vi "MRay Auton.vi"(0 "Auton Array":dbl[][](array[numeric])) -> (13 "Shooter":dbl, 14 "Left Drive":dbl, 15 "Right Drive":dbl, 16 "Ramp ACT motor":dbl, 17 "Conveyor":dbl, 18 "Harvester":dbl, 19 "Turret Rotation":dbl)   [LabVIEW 2011]
uses:
  Robot Global Data.vi
panel:
  out "Tzero":i64
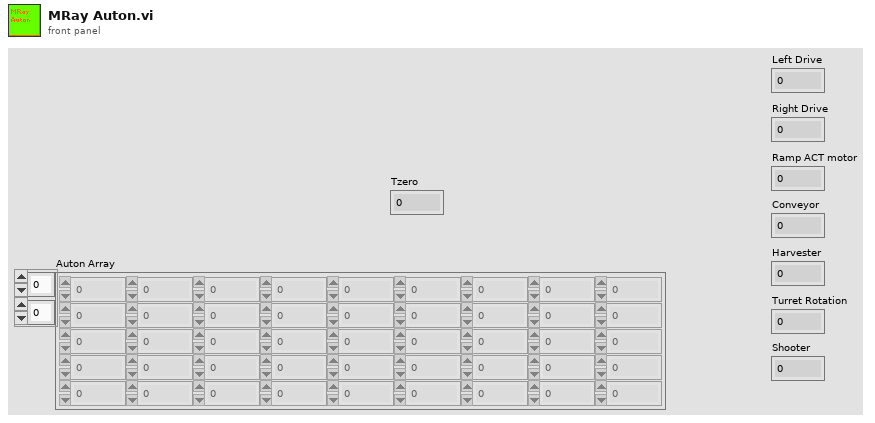
[diagram p1: front panel]
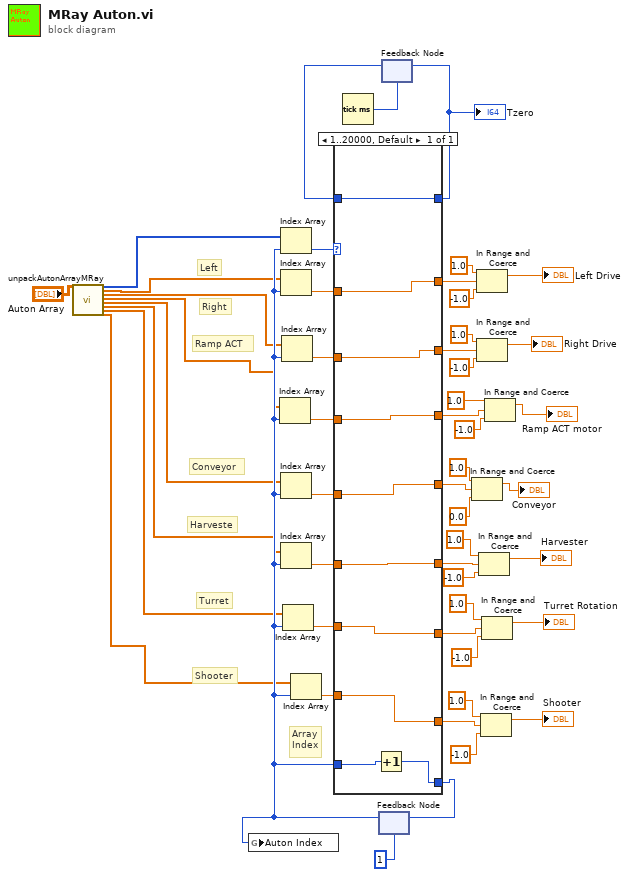
[diagram p0: block diagram]
diagram:
  # "Array\nIndex"
  # "Ramp ACT"
  # "Right"
  # "Left"
  # "Conveyor"
  # "Harveste"
  # "Turret"
  # "Shooter"
  n1 = call "unpackAutonArrayMRay.vi"("all rows"="Auton Array") -> ("Primitive"=w28:i16[], "Left Drive"=w7:dbl[], "Right Drive"=w6:dbl[], "Ramp ACT"=w5:dbl[], "Conveyor"=w4:dbl[], "Harvester"=w3:dbl[], "Turret"=w2:dbl[], "Shooter"=w1:dbl[])  [unwired: 19 in]
  n2 = Tick Count (ms)() -> (millisecond timer value=w49:u32)
  n3 = feedback #1(1) -> (w26:i32)
  n4 = global write "Robot Global Data.vi" "Auton Index"(w26) -> ()
  n5 = Index Array(array=w5, index=w26) -> (element=w16:dbl)
  n6 = Index Array(array=w28, index=w26) -> (element=w27:i16)
  n7 = Index Array(array=w7, index=w26) -> (element=w20:dbl)
  n8 = Index Array(array=w4, index=w26) -> (element=w14:dbl)
  n9 = Index Array(array=w3, index=w26) -> (element=w12:dbl)
  n10 = Index Array(array=w6, index=w26) -> (element=w18:dbl)
  n11 = Index Array(array=w2, index=w26) -> (element=w10:dbl)
  n12 = Index Array(array=w1, index=w26) -> (element=w8:dbl)
  n13 = feedback #2(w49) -> (w50:u32)
  n14 = case shown="1..20000, Default" w27 {
    tunnel: [w61] -> w42
    tunnel: w50 -> [w61]
    tunnel: w26 -> [w60]
    tunnel: [w59] -> w22
    tunnel: [w58] -> w21
    tunnel: w20 -> [w58]
    tunnel: [w57] -> w19
    tunnel: w18 -> [w57]
    tunnel: [w56] -> w17
    tunnel: w16 -> [w56]
    tunnel: [w55] -> w15
    tunnel: w14 -> [w55]
    tunnel: [w54] -> w13
    tunnel: w12 -> [w54]
    tunnel: [w53] -> w11
    tunnel: w10 -> [w53]
    tunnel: [w52] -> w9
    tunnel: w8 -> [w52]
    frame 1..20000, Default {
      n15 = Increment(x=w60) -> (x+1=w59:i32)
    }
  }
  "Tzero" <- w42
  n16 = feedback-in #1(w22) -> ()
  n17 = feedback-in #2(w42) -> ()
  n18 = In Range and Coerce(upper limit=1.0, x=w15, lower limit=0.0) -> (coerced(x)=→"Conveyor":dbl)  [unwired: 1 out]
  n19 = In Range and Coerce(upper limit=1.0, x=w21, lower limit=-1.0) -> (coerced(x)=→"Left Drive":dbl)  [unwired: 1 out]
  n20 = In Range and Coerce(upper limit=1.0, x=w19, lower limit=-1.0) -> (coerced(x)=→"Right Drive":dbl)  [unwired: 1 out]
  n21 = In Range and Coerce(upper limit=1.0, x=w13, lower limit=-1.0) -> (coerced(x)=→"Harvester":dbl)  [unwired: 1 out]
  n22 = In Range and Coerce(upper limit=1.0, x=w9, lower limit=-1.0) -> (coerced(x)=→"Shooter":dbl)  [unwired: 1 out]
  n23 = In Range and Coerce(upper limit=1.0, x=w11, lower limit=-1.0) -> (coerced(x)=→"Turret Rotation":dbl)  [unwired: 1 out]
  n24 = In Range and Coerce(upper limit=1.0, x=w17, lower limit=-1.0) -> (coerced(x)=→"Ramp ACT motor":dbl)  [unwired: 1 out]
